vi "MAT_HB0_filter.vi"(1 "HB smoothing filter coefficients (exact up to x^4)":dbl[](array[numeric])=[-0.0625, 0.25, 0.625, 0.25, -0.0625], 2 "N samples":i32, 3 "Input sample":dbl) -> (0 "Filtered sample":dbl)   [LabVIEW 2018, in "Tracker.lvlib"]
uses:
  Tracker.lvlib
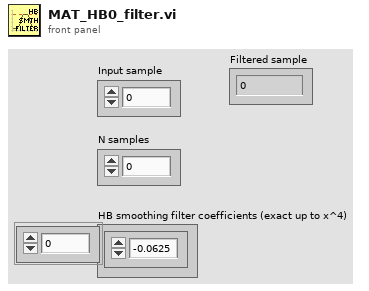
[diagram p1: front panel]
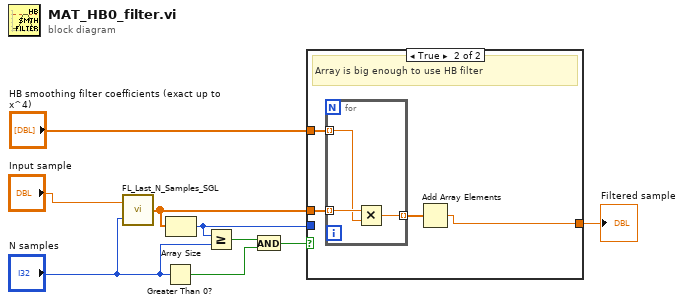
[diagram p0: block diagram]
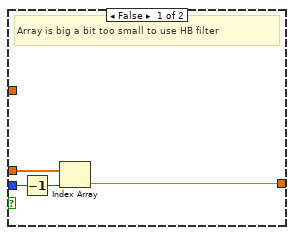
[diagram p2: hidden frame]
diagram:
  n1 = call "FL_Last_N_Samples_SGL.vi"("BufferLengthSamples"="N samples", "Input sample"="Input sample") -> ("Output Array"=w9:dbl[])
  n2 = Greater Than 0?(x="N samples") -> (x > 0?=w5:bool)
  n3 = Array Size(array=w9) -> (size(s)=w8:i32)
  n4 = Greater Or Equal?(x=w8, y="N samples") -> (x >= y?=w6:bool)
  n5 = And(x=w6, y=w5) -> (x .and. y?=w7:bool)
  n6 = case shown="True" w7 {
    tunnel: w9 -> [w13 w17]
    tunnel: "HB smoothing filter coefficients (exact up to x^4)" -> [_ w16]
    tunnel: [w12 w14] -> w1
    tunnel: w8 -> [w11 _]
    frame False {
      # "Array is big a bit too small to use HB filter"
      n7 = Decrement(x=w11) -> (x-1=w10:i32)
      n8 = Index Array(array=w13, index=w10) -> (element=w12:dbl)
    }
    frame True {
      # "Array is big enough to use HB filter"
      n9 = for {
        tunnel: w17 -> [w20] mode=indexing
        tunnel: w16 -> [w18] mode=indexing
        tunnel: [w19] -> w15 mode=indexing
        n10 = Multiply(x=w20, y=w18) -> (x*y=w19:dbl)
      }
      n11 = Add Array Elements(numeric array=w15) -> (sum=w14:dbl)
    }
  }
  "Filtered sample" <- w1
